vi "Delete Splash Screen User Event.vi"(8 "error in (no error)":errorcluster) -> (0 "error out":errorcluster)   [LabVIEW 2016, in "SLL Splash Screen.lvlib"]
uses:
  SLL Splash Screen.lvlib
  _Typedefs/User Event LV2 Command.ctl
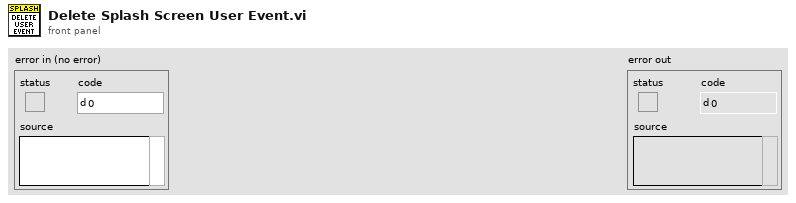
[diagram p1: front panel]
types:
  T1 = typedef "SLL Splash Screen.lvlib/User Event LV2 Command.ctl" = enum16{"Create", "Generate", "Delete"}
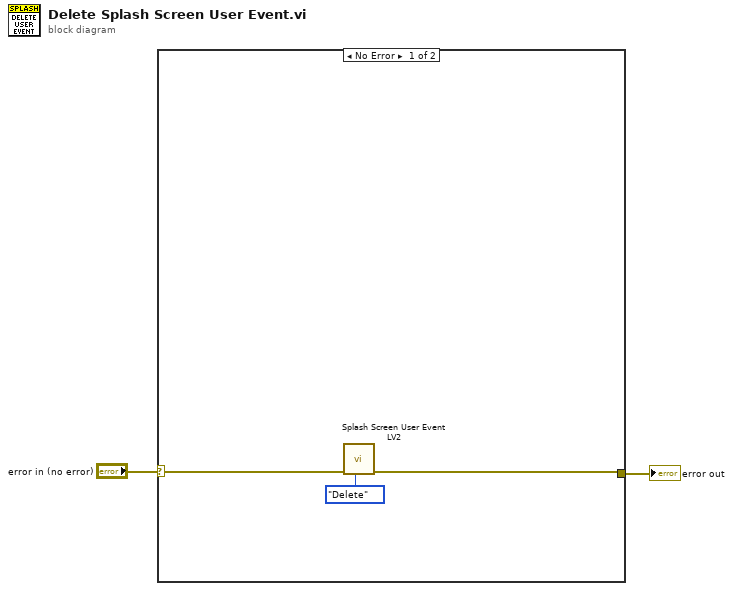
[diagram p0: block diagram]
diagram:
  n1 = case shown="No Error" "error in (no error)" {
    selector: "error in (no error)" -> [w5 w6]
    tunnel: [w4 w6] -> w1
    frame No Error {
      n2 = call "Splash Screen User Event LV2.vi"("Command"=User_Event_LV2_Command."Delete", "error in (no error)"=w5) -> ("error out"=w4:errorcluster)  [unwired: 8 in, 1 out]
    }
    frame Error {
    }
  }
  "error out" <- w1
